vi "RSZVB Configure Pulse Generators.vi"(6 "Ext Signal Generator Output (Off)":bool, 7 "Assignment (0)":i32(ring) items=["Gen 1 Controls All Modulators", "Gen 2 Controls All Modulators", "Gen 1 Controls Modulators 1 And 3, Gen 2 Controls Modulator 2", "Gen 1 Controls Modulators 1 And 2, Gen 2 Controls Modulator 3"], 8 "error in (no error)":errorcluster {"code" format="%.0x"}, 9 "Ext Signal Generator Input (Off)":bool, 10 "Channel (1)":i32=1, 11 "VISA session":refnum<visa-resource-name>) -> (0 "error out":errorcluster {"code" format="%.0x"}, 3 "dup VISA session":refnum<visa-resource-name>)   [LabVIEW 2011]
doc: "This VI defines the source and the output of the pulse generator signals and assigns pulse generator signals to the pulse modulators of the Extension Unit R&S ZVAXxx.\n\nRemote-control command(s):\n[SENSe<Ch>:]EUNit:PGENerator:INPut:EXTernal\n[SENSe<Ch>:]EUNit:PGENerator:ASSignment G1Mall | G2Mall | G1M2 | G1M3\n[SENSe<Ch>:]EUNit:PGENerator:OUTPut:EXTernal"
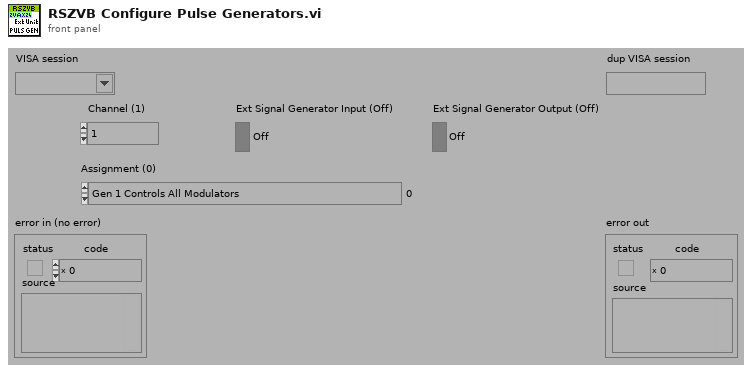
[diagram p1: front panel]
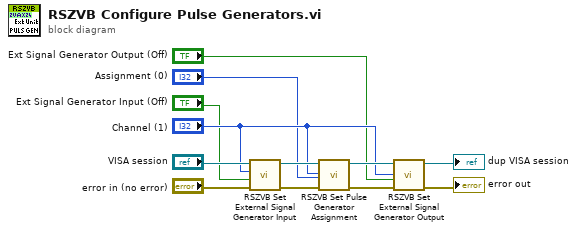
[diagram p0: block diagram]
diagram:
  n1 = call "RSZVB Set External Signal Generator Input.vi"("error in (no error)"="error in (no error)", "Ext Signal Generator Input (Off)"="Ext Signal Generator Input (Off)", "Channel (1)"="Channel (1)", "VISA session"="VISA session") -> ("error out"=w10:errorcluster, "dup VISA session"=w9:refnum<visa-resource-name>)  [unwired: 6 in]
  n2 = call "RSZVB Set Pulse Generator Assignment.vi"("error in (no error)"=w10, "Assignment (0)"="Assignment (0)", "Channel (1)"="Channel (1)", "VISA session"=w9) -> ("error out"=w8:errorcluster, "dup VISA session"=w7:refnum<visa-resource-name>)  [unwired: 6 in]
  n3 = call "RSZVB Set External Signal Generator Output.vi"("error in (no error)"=w8, "Ext Signal Generator Output (Off)"="Ext Signal Generator Output (Off)", "Channel (1)"="Channel (1)", "VISA session"=w7) -> ("error out"=→"error out":errorcluster, "dup VISA session"=→"dup VISA session":refnum<visa-resource-name>)  [unwired: 6 in]
